vi "Print Py Object.vi"(8 "error in (no error)":errorcluster, 10 "Python Object Refnum in":T1, 11 "Session Handle in":refnum<data-value>) -> (0 "error out":errorcluster, 1 "Print Ouptut":string, 2 "Python Object Refnum out":T1, 3 "Session Handle out":refnum<data-value>)   [LabVIEW 2020, in "G-Embedded-Python-Interpreter-Toolkit.lvlib"]
uses:
  G-Embedded-Python-Interpreter-Toolkit.lvlib
  Python Object Reference.ctl
  Python Object Type.ctl
  bin/gepit.cp310.32.dll
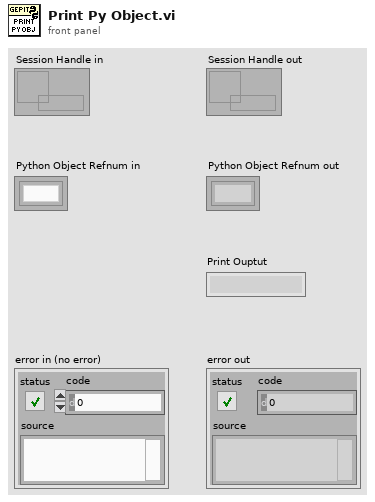
[diagram p1: front panel]
types:
  T1 = typedef "G-Embedded-Python-Interpreter-Toolkit.lvlib/Python Object Reference.ctl" = refnum<k1>
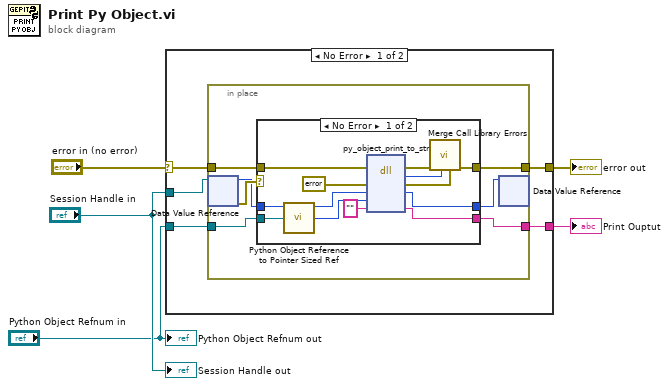
[diagram p0: block diagram]
diagram:
  n1 = case shown="No Error" "error in (no error)" {
    selector: "error in (no error)" -> [w9 w32]
    tunnel: "Session Handle in" -> [w10 _]
    tunnel: [w8 w32] -> w4
    tunnel: "Python Object Refnum in" -> [w7 _]
    tunnel: [w6 _] -> w1
    frame No Error {
      n2 = in-place {
        in-place-border: w9 -> [w16]
        in-place-border: [w13] -> w8
        in-place-border: w7 -> [w12]
        in-place-border: [w11] -> w6
        n3 = in-place-dvr #1(w10) -> (w15:u64, w17:errorcluster)
        n4 = case shown="No Error" w17 {
          selector: w17 -> [_ w30]
          tunnel: w16 -> [w25 _]
          tunnel: w15 -> [w24 w31]
          tunnel: [w23 w31] -> w14
          tunnel: [w22 w30] -> w13
          tunnel: w12 -> [w21 _]
          tunnel: [w20 _] -> w11
          frame No Error {
            n5 = call "Python Object Reference to Pointer Sized Ref.vi"("Refnum in"=w21) -> ("Py Object"=w18:u64)
            n6 = dll-call lib="C:/serenial/libraries/g-embedded-python-interpreter-toolkit/LabVIEW/bin/gepit.cp310.32.dll" fn="py_object_print_to_str"(error in=w25, "Error"=errorcluster {"status"=FALSE, "code"=0, "source"=""} ("error constant"), "Session"=w24, "Py Object"=w18, "Value"="") -> (error out=w28:errorcluster, "return type"=w27:i32, "Error"=w26:errorcluster, "Session"=w23:u64, "Value"=w20:string)  [unwired: 3 in, 1 out]
            n7 = call "Merge Call Library Errors.vi"("Call Library Error"=w26, "Return Value"=w27, "error in"=w28) -> ("error out"=w22:errorcluster)  [unwired: 8 in]
          }
          frame Error {
          }
        }
        n8 = in-place-dvr #1(w14) -> ()  [unwired: 2 out]
      }
    }
    frame Error {
    }
  }
  "error out" <- w4
  "Print Ouptut" <- w1
  "Session Handle out" <- "Session Handle in"
  "Python Object Refnum out" <- "Python Object Refnum in"
